vi "GT Set Axis Band.vi"(7 "time":i32, 8 "error in (no error)":errorcluster caption="错误输入（无错误）", 9 "band":i32, 10 "axis":i16, 11 "cardNum":i16) -> (0 "error out":errorcluster caption="错误输出", 3 "function return":i16)   [LabVIEW 2014, in "gts.lvlib"]
doc: "GT_API GT_SetAxisBand(short cardNum,short axis,long band,long time);"
uses:
  gts.lvlib
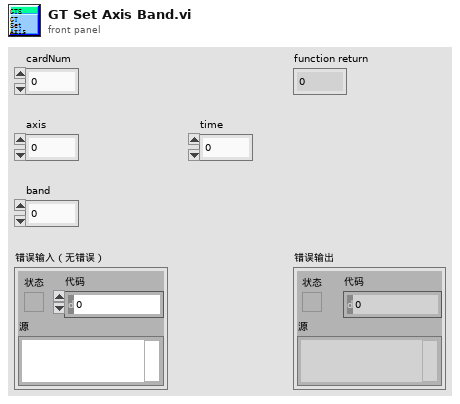
[diagram p1: front panel]
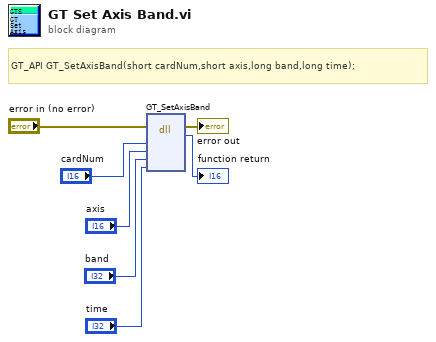
[diagram p0: block diagram]
diagram:
  # "GT_API GT_SetAxisBand(short cardNum,short axis,long band,long time);"
  n1 = dll-call lib="PTH2habs D固高科技资料GTS控制卡GTS卡18年上半年资料dllVC32bit\nmulti_cardgts.*" fn="GT_SetAxisBand"(error in="error in (no error)", "cardNum"="cardNum", "axis"="axis", "band"="band", "time"="time") -> (error out=→"error out":errorcluster, →"function return":i16)  [unwired: 6 in, 1 out]
